vi "Part 1.vi"(11 "Input":string) -> (3 "Output":i64)   [LabVIEW 2021]
uses:
  <userlib>/_OpenG.lib/string/string.llb/Convert EOLs (String)__ogtk.vi
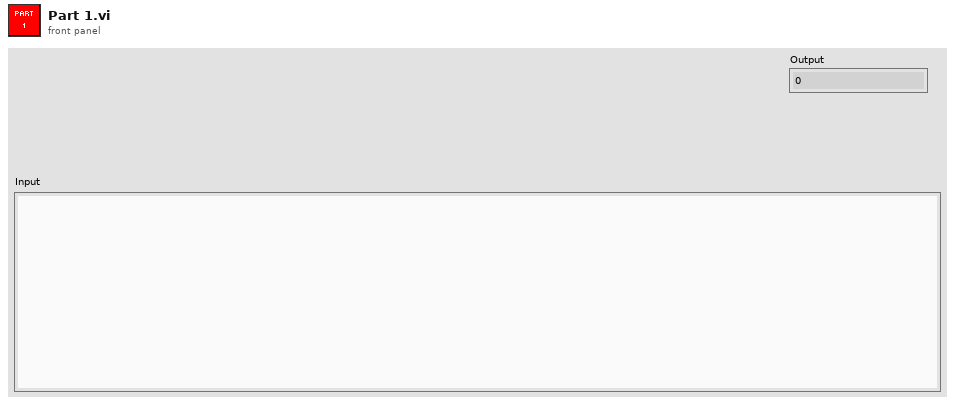
[diagram p1: front panel]
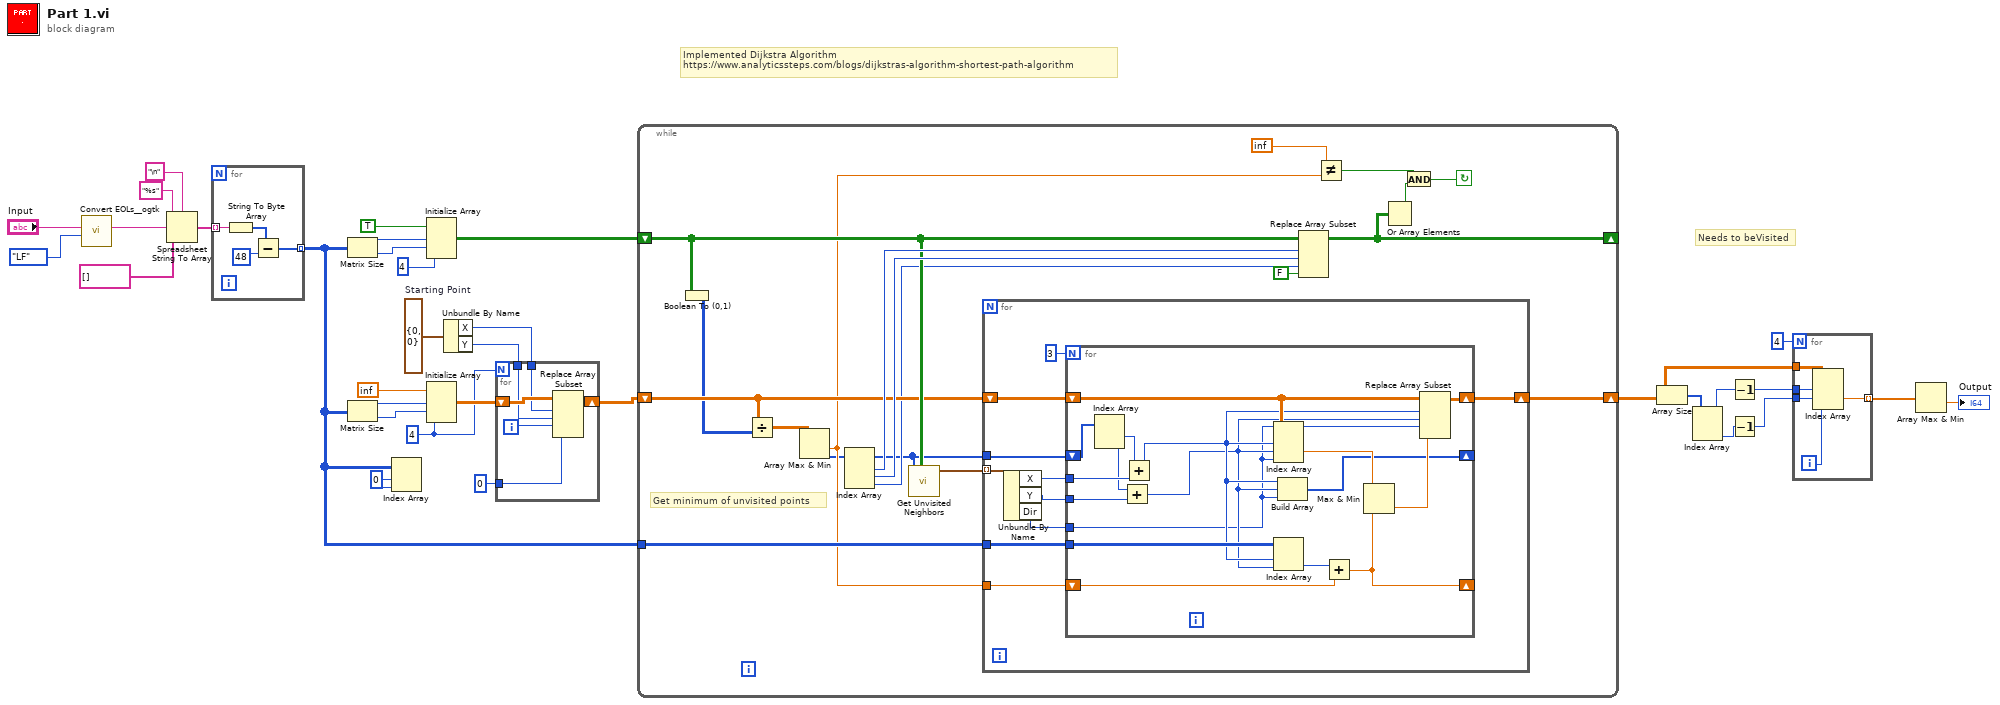
[diagram p0: block diagram]
diagram:
  w3 = 0 ("index (row)")
  w5 = 4
  w19 = cluster{"X":i32, "Y":i32} {"X"=0, "Y"=0}  # Starting Point
  # "Implemented Dijkstra Algorithm\nhttps://www.analyticssteps.com/blogs/dijkstras-algorithm-shortest-path-algorithm"
  # "Needs to beVisited"
  n1 = call-poly <userlib>:"Convert EOLs__ogtk.vi"("Convert to:"=enum16{"CR", "LF", "CRLF"}."LF", "String in"="Input") -> ("String out"=w29:string)  [unwired: 9 in]
  n2 = Spreadsheet String To Array(delimiter (Tab)="\n", format string="%s", spreadsheet string=w29, array type (2D Dbl)=string[] []) -> (array=w27:string[])
  n3 = for {
    tunnel: w27 -> [w37] mode=indexing
    tunnel: [w34] -> w4 mode=indexing
    n4 = String To Byte Array(string=w37) -> (unsigned byte array=w36:u8[])
    n5 = Subtract(x=w36, y=u8 48) -> (x-y=w34:u8[])
  }
  n6 = Matrix Size(0:w4) -> (1:w26:i32, 2:w12:i32)
  n7 = Matrix Size(0:w4) -> (1:w22:i32, 2:w13:i32)
  n8 = Index Array(array=w4, index (row)=w3, index (col)=w3) -> ()  [unwired: 1 out]
  n9 = Initialize Array(TRUE, w26, w12, 4) -> (w24:bool[][][])
  n10 = Initialize Array(inf, w22, w13, w5) -> (w23:dbl[][][])
  n11 = Unbundle By Name(w19) -> ("X"=w17:i32, "Y"=w18:i32)
  n12 = for {
    N: w5 -> [_]
    tunnel: w18 -> [w41]
    tunnel: w17 -> [w40]
    shift-right: [w42] -> w20
    shift-left: w23 -> [w43]
    tunnel: u8 0 -> [w38]
    i -> [w39]
    n13 = Replace Array Subset(array=w43, new element=w38, index (dim 0)=w40, index (dim 1)=w41, index (dim 2)=w39) -> (w42:dbl[][][])
  }
  n14 = while {
    shift-right: [w56] -> _
    shift-left: w24 -> [w54]
    shift-right: [w59] -> w15
    shift-left: w20 -> [w53]
    tunnel: w4 -> [w60]
    stop <- w48 continue-if-true
    # "Get minimum of unvisited points"
    n15 = Boolean To (0,1)(Boolean=w54) -> (0, 1=w52:i16[][][])
    n16 = Divide(x=w53, y=w52) -> (x/y=w51:dbl[][][])
    n17 = Array Max & Min(array=w51) -> (min value=w45:dbl, min index (indices)=w44:i32[])  [unwired: 2 out]
    n18 = Index Array(array=w44) -> (element #1=w58:i32, element #2=w57:i32, element #3=w50:i32)  [unwired: 3 in]
    n19 = call "Get Unvisited Neighbors.vi"("Unvisited"=w54, "Current Point"=w44) -> ("Unvisited Neighbors"=w55:cluster{"X":i32, "Y":i32, "Dir":i32}[])  [unwired: 9 in]
    n20 = for {
      tunnel: w60 -> [w71]
      tunnel: w55 -> [w65] mode=indexing
      tunnel: w45 -> [w68]
      shift-right: [w70] -> w59
      shift-left: w53 -> [w69]
      tunnel: w44 -> [w66]
      n21 = Unbundle By Name(w65) -> ("X"=w64:i32, "Y"=w63:i32, "Dir"=w62:i32)
      n22 = for {
        N: 3 -> [_]
        shift-right: [w85] -> w70
        shift-left: w69 -> [w86]
        tunnel: w71 -> [w84]
        shift-right: [w82] -> _
        shift-left: w68 -> [w88]
        shift-right: [w72] -> _
        shift-left: w66 -> [w80]
        tunnel: w64 -> [w78]
        tunnel: w63 -> [w76]
        tunnel: w62 -> [w73]
        n23 = Index Array(array=w80) -> (element #1=w79:i32, element #2=w77:i32)  [unwired: 2 in]
        n24 = Add(x=w77, y=w76) -> (x+y=w74:i32)
        n25 = Add(x=w79, y=w78) -> (x+y=w75:i32)
        n26 = Index Array(array=w86, index (dim 0)=w75, index (dim 1)=w74, index (dim 2)=w73) -> (element=w87:dbl)
        n27 = Index Array(array=w84, index (row)=w75, index (col)=w74) -> (element=w83:u8)
        n28 = Build Array(w75, w74, w73) -> (w72:i32[])
        n29 = Add(x=w83, y=w88) -> (x+y=w82:dbl)
        n30 = Max & Min(x=w87, y=w82) -> (min(x,y)=w81:dbl)  [unwired: 1 out]
        n31 = Replace Array Subset(array=w86, new element=w81, index (dim 0)=w75, index (dim 1)=w74, index (dim 2)=w73) -> (w85:dbl[][][])
      }
    }
    n32 = Replace Array Subset(array=w54, new element=FALSE, index (dim 0)=w58, index (dim 1)=w57, index (dim 2)=w50) -> (w56:bool[][][])
    n33 = Not Equal?(x=inf, y=w45) -> (x != y?=w46:bool)
    n34 = Or Array Elements(Boolean array=w56) -> (logical OR=w49:bool)
    n35 = And(x=w46, y=w49) -> (x .and. y?=w48:bool)
  }
  n36 = Array Size(array=w15) -> (size(s)=w10:i32[])
  n37 = Index Array(array=w10) -> (element #1=w9:i32, element #2=w8:i32)  [unwired: 2 in]
  n38 = Decrement(x=w9) -> (x-1=w16:i32)
  n39 = Decrement(x=w8) -> (x-1=w11:i32)
  n40 = for {
    N: 4 -> [_]
    tunnel: w16 -> [w93]
    tunnel: w15 -> [w92]
    tunnel: [w91] -> w14 mode=indexing
    tunnel: w11 -> [w90]
    i -> [w89]
    n41 = Index Array(array=w92, index (dim 0)=w93, index (dim 1)=w90, index (dim 2)=w89) -> (element=w91:dbl)
  }
  n42 = Array Max & Min(array=w14) -> (min value=→"Output":dbl)  [unwired: 3 out]
